vi "Read XML HW Configuration File_Extra Checks_Check Label Name Uniqueness For Each hardWareChannel.vi"(8 "error in (no error)":errorcluster, 11 "Array In":T1[](array[typedef]) {"speed" items=["Auto", "Low", "High"]; "Labels"."scheduleBuildUnit" items=["Millisecond", "Microsecond"]}) -> (0 "error out":errorcluster)   [LabVIEW 2020]
doc: "This VI checks that for a given Hardware Channel, each Label Name is unique."
uses:
  Controls/Ballard_Channel.ctl
  Controls/Ballard_Label.ctl
  Controls/Ballard_Word.ctl
  Controls/ARINCParam.ctl
  Shared/Controls and Global/TransferType.ctl
  Controls/Channel_direction.ctl
  Controls/Channel Speed.ctl
  <userlib>/_OpenG.lib/md5/md5.llb/MD5 Message Digest (Binary String)__ogtk.vi
  <userlib>/_OpenG.lib/array/array.llb/Remove Duplicates from 1D Array (String)__ogtk.vi
  Shared/Ballard Arinc-429 Shared.lvlib
  Ballard Arinc-429 System Explorer.lvlib
panel:
  out "Error Source":string
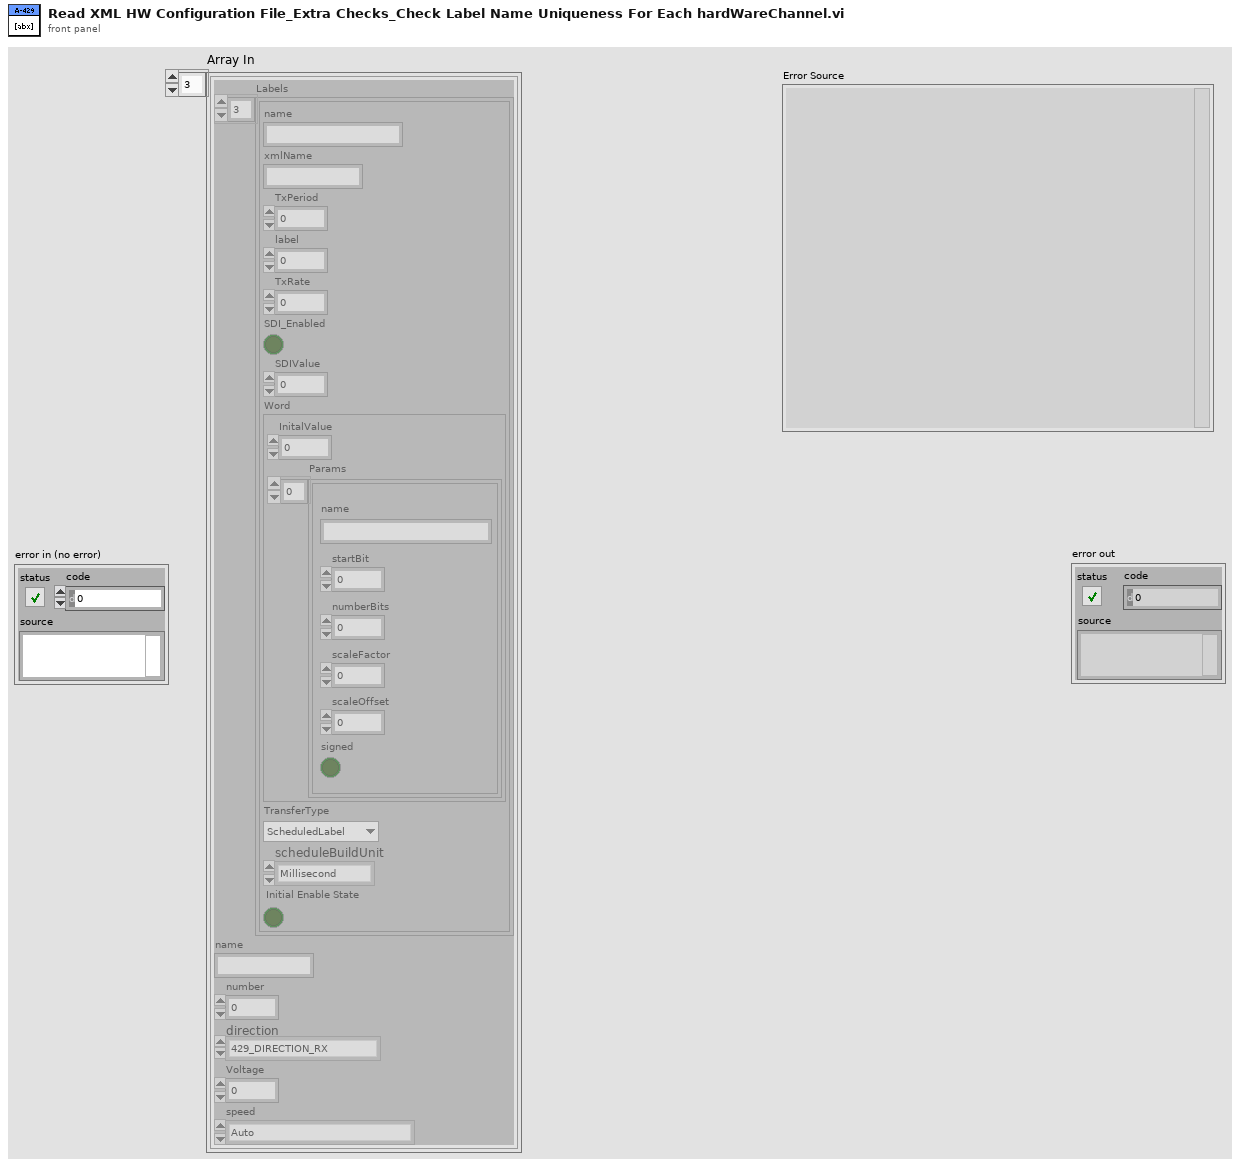
[diagram p1: front panel]
types:
  T1 = typedef "Ballard Arinc-429 System Explorer.lvlib/Ballard_Channel.ctl" = cluster{"Labels":T2[], "name":string, "number":u8, "direction":T6, "Voltage":dbl, "speed":T7}
  T2 = typedef "Ballard Arinc-429 System Explorer.lvlib/Ballard_Label.ctl" = cluster{"name":string, "xmlName":string, "TxPeriod":u32, "label":u32, "TxRate":dbl, "SDI_Enabled":bool, "SDIValue":u8, "Word":T3, "TransferType":T5, "scheduleBuildUnit":i32, "Initial Enable State":bool}
  T3 = typedef "Ballard Arinc-429 System Explorer.lvlib/Ballard_Word.ctl" = cluster{"InitalValue":u32, "Params":T4[]}
  T4 = typedef "Ballard Arinc-429 System Explorer.lvlib/ARINCParam.ctl" = cluster{"name":string, "startBit":i32, "numberBits":i32, "scaleFactor":dbl, "scaleOffset":dbl, "signed":bool}
  T5 = typedef "Ballard Arinc-429 Shared.lvlib/TransferType.ctl" = enum16{"ScheduledLabel", "Acyclic", "Block", "Strobe"}
  T6 = typedef "Ballard Arinc-429 System Explorer.lvlib/Channel_direction.ctl" = enum16{"429_DIRECTION_RX", "429_DIRECTION_TX"}
  T7 = typedef "Ballard Arinc-429 System Explorer.lvlib/Channel Speed.ctl" = i32
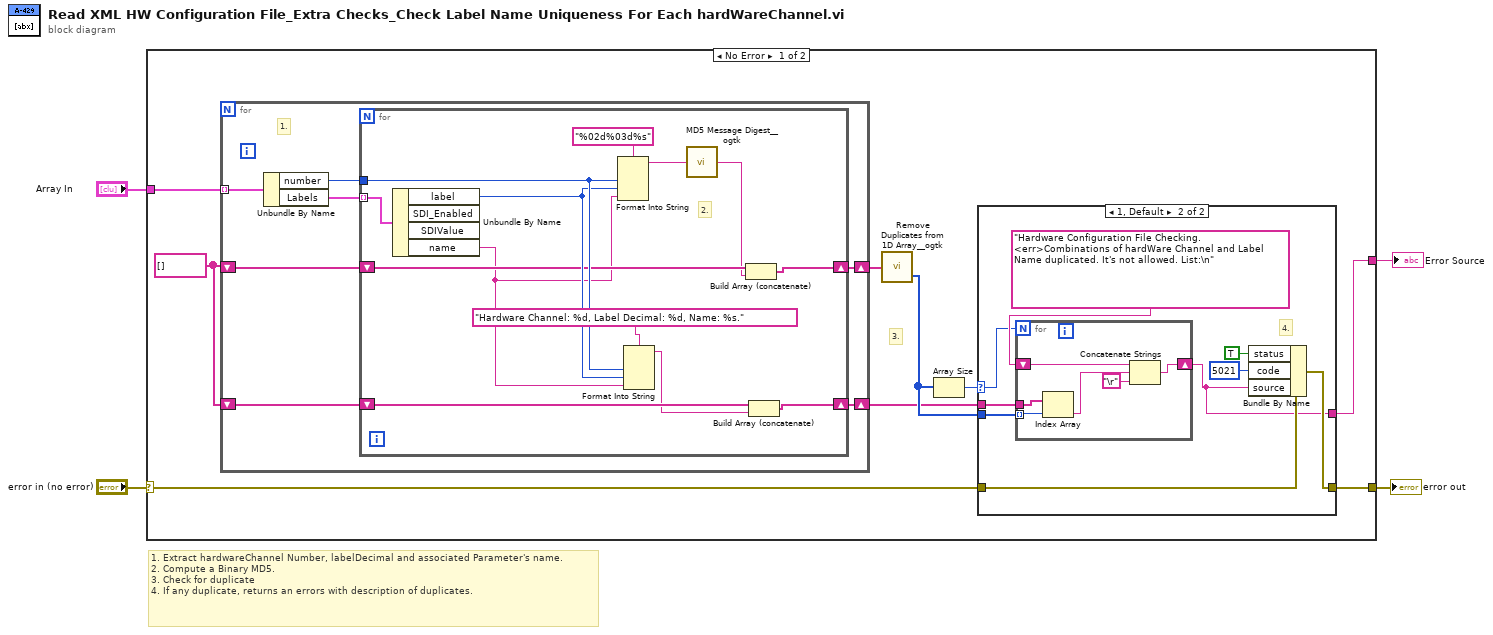
[diagram p0: block diagram]
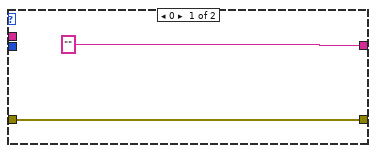
[diagram p2: hidden frame]
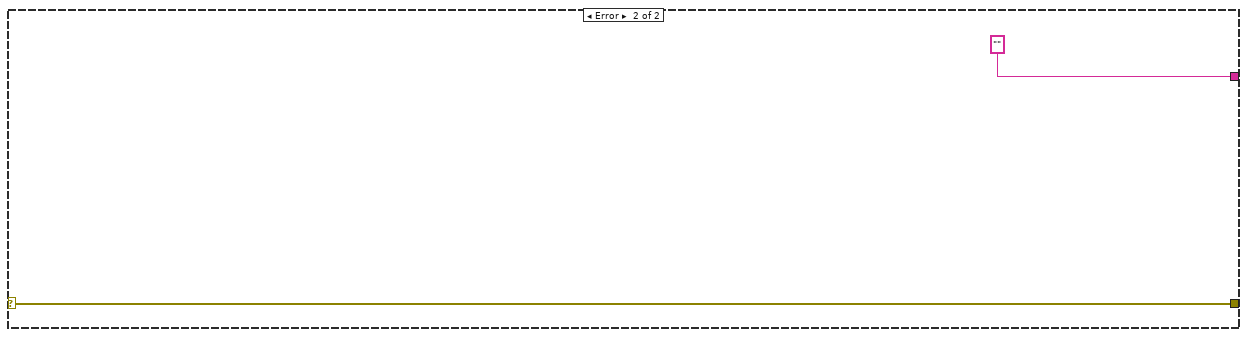
[diagram p3: hidden frame]
diagram:
  # "1. Extract hardwareChannel Number, labelDecimal and associated Parameter's name.\n2. Compute a Binary MD5.\n3. Check for duplicate\n4. If any duplicate, returns an errors with description of duplicates."
  n1 = case shown="No Error" "error in (no error)" {
    selector: "error in (no error)" -> [w12 w52]
    tunnel: [w9 w52] -> w3
    tunnel: "Array In" -> [w11 _]
    tunnel: [w8 ""] -> w1
    frame No Error {
      w6 = string[] []
      # "3."
      n2 = for {
        tunnel: w11 -> [w37] mode=indexing
        shift-right: [w33] -> w7
        shift-left: w6 -> [w34]
        shift-right: [w31] -> w5
        shift-left: w6 -> [w32]
        # "1."
        n3 = Unbundle By Name(w37) -> ("number"=w36:u8, "Labels"=w35:T2[])
        n4 = for {
          tunnel: w36 -> [w50]
          tunnel: w35 -> [w49] mode=indexing
          shift-right: [w46] -> w33
          shift-left: w34 -> [w47]
          shift-right: [w44] -> w31
          shift-left: w32 -> [w45]
          # "2."
          n5 = Unbundle By Name(w49) -> ("label"=w48:u32, "name"=w38:string)  [unwired: 2 out]
          n6 = Format Into String(format string="%02d%03d%s", w50, w48, w38) -> (resulting string=w42:string)  [unwired: 2 in, 1 out]
          n7 = Format Into String(format string="Hardware Channel: %d, Label Decimal: %d, Name: %s.", w50, w48, w38) -> (resulting string=w39:string)  [unwired: 2 in, 1 out]
          n8 = call-poly <userlib>:"MD5 Message Digest__ogtk.vi"("Message"=w42) -> ("MD5 Message Digest"=w41:string)
          n9 = Build Array (concatenate)(w47, w41) -> (w46:string[])
          n10 = Build Array (concatenate)(w45, w39) -> (w44:string[])
        }
      }
      n11 = call-poly <userlib>:"Remove Duplicates from 1D Array__ogtk.vi"("Input Array"=w7) -> ("indices of removed elements"=w10:i32[])  [unwired: 1 out]
      n12 = Array Size(array=w10) -> (size(s)=w13:i32)
      n13 = case shown="1, Default" w13 {
        selector: w13 -> [_ w19]
        tunnel: w12 -> [w15 w24]
        tunnel: w10 -> [_ w18]
        tunnel: [w15 w23] -> w9
        tunnel: ["" w17] -> w8
        tunnel: w5 -> [_ w16]
        frame 0 {
        }
        frame 1, Default {
          # "4."
          n14 = for {
            N: w19 -> [_]
            shift-right: [w29] -> w17
            shift-left: "Hardware Configuration File Checking.<err>Combinations of hardWare Channel and Label Name duplicated. It's not allowed. List:\n" -> [w30]
            tunnel: w18 -> [w28] mode=indexing
            tunnel: w16 -> [w26]
            n15 = Index Array(array=w26, index=w28) -> (element=w25:string)
            n16 = Concatenate Strings(w30, w25, "\r") -> (w29:string)
          }
          n17 = Bundle By Name(cluster=w24, "status"=TRUE, "code"=5021, "source"=w17) -> (w23:errorcluster)
        }
      }
    }
    frame Error {
    }
  }
  "error out" <- w3
  "Error Source" <- w1
